vi "Wait.vi"(8 "error in (no error)":errorcluster, 10 "Timeout":i32=1000, 11 "HAMAMATSU_DCAMAPI in":refnum<class "HAMAMATSU_DCAMAPI.lvclass">) -> (0 "error out":errorcluster, 3 "HAMAMATSU_DCAMAPI out":refnum<class "HAMAMATSU_DCAMAPI.lvclass">)   [LabVIEW 2020, in "HAMAMATSU_DCAMAPI.lvclass"]
uses:
  HAMAMATSU_DCAMAPI.lvclass
  HAMAMATSU_DCAMAPI.lvclass/HAMAMATSU_DCAMAPI.ctl
panel:
  out "Frame Count":i32
  out "Frame Index":i32
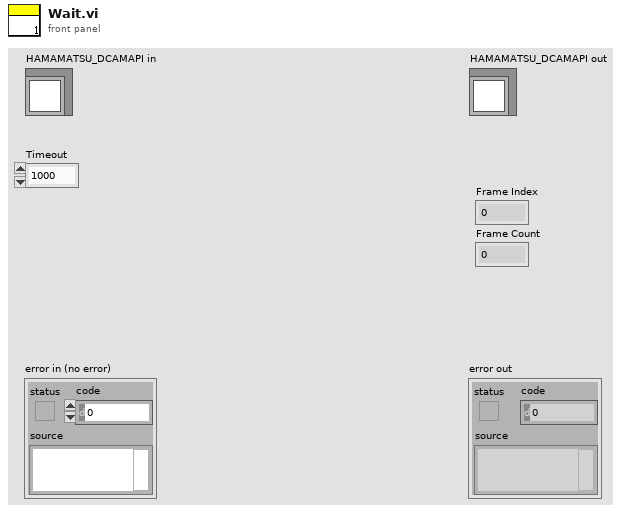
[diagram p1: front panel]
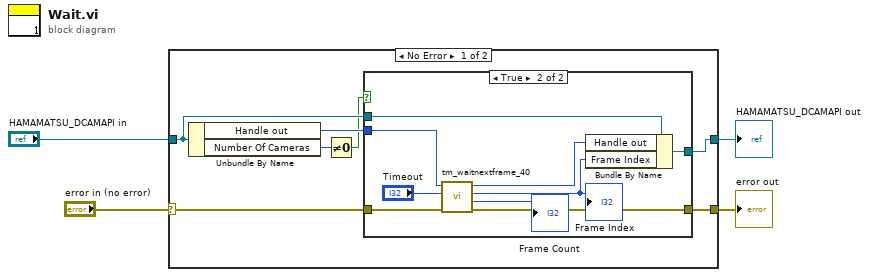
[diagram p0: block diagram]
diagram:
  n1 = case shown="No Error" "error in (no error)" {
    selector: "error in (no error)" -> [w11 w24]
    tunnel: "HAMAMATSU_DCAMAPI in" -> [w8 w23]
    tunnel: [w10 w24] -> w2
    tunnel: [w9 w23] -> w1
    frame No Error {
      n2 = Unbundle By Name(w8) -> ("Handle out"=w7:u32, "Number Of Cameras"=w6:u32)
      n3 = Not Equal To 0?(x=w6) -> (x != 0?=w5:bool)
      n4 = case shown="True" w5 {
        tunnel: w11 -> [w12 w22]
        tunnel: [w12 w21] -> w10
        tunnel: w8 -> [w13 w18]
        tunnel: [w13 w17] -> w9
        tunnel: w7 -> [_ w19]
        frame False {
        }
        frame True {
          n5 = call <userlib>:"tm_waitnextframe_40.vi"("error in (no error)"=w22, "Timeout"="Timeout", "Handle in"=w19) -> ("error out"=w21:errorcluster, "Frame Count"=→"Frame Count":i32, "Frame Index"=w16:i32, "Handle out"=w15:u32)  [unwired: 5 in]
          "Frame Index" <- w16
          n6 = Bundle By Name(cluster=w18, "Handle out"=w15, "Frame Index"=w16) -> (w17:refnum<class "HAMAMATSU_DCAMAPI.lvclass">)
        }
      }
    }
    frame Error {
    }
  }
  "error out" <- w2
  "HAMAMATSU_DCAMAPI out" <- w1
